vi "UndoEngine.vi"(0 "reference":refnum<class "Graph.lvclass">, 1 "Action":enum16{"TakeSnapshot", "Undo", "Redo"}(ring), 2 "Reset":bool, 3 "graphics":refnum<class "Graphics.lvclass">, 4 "grid":refnum<class "Grid.lvclass">, 5 "error in (no error)":errorcluster, 6 "menu":refnum<k9>, 8 "UndoLevels(ignoredIfNotWired)":i32=-1) -> (19 "error out":errorcluster)   [LabVIEW 2014, in "Graph.lvclass"]
doc: "Save to File"
uses:
  <resource>/Framework/Providers/Open_GDS/UML/Graph_class/Graph.lvclass
  <resource>/Framework/Providers/Open_GDS/UML/Grid_class/Grid.lvclass
  <resource>/Framework/Providers/Open_GDS/UML/Graphics_class/Graphics.lvclass
  <resource>/Framework/Providers/Open_GDS/UML/Graph_class/private/diagramType.ctl
  <resource>/Framework/Providers/Open_GDS/UML/AbstractNode_class/AbstractNode.lvclass
  <resource>/Framework/Providers/Open_GDS/UML/AbstractEdge_class/AbstractEdge.lvclass
  <resource>/Framework/Providers/Open_GDS/UML/General/Rectangle/Rectangle Rectangle2D.ctl
  <resource>/Framework/Providers/Open_GDS/UML/StateDiagramGraph_class/private/StateDiagramData.ctl
  <resource>/Framework/Providers/Open_GDS/UML/StateDiagramGraph_class/private/ViPathShowOption.ctl
  <resource>/Framework/Providers/Open_GDS/UML/ClassDiagramGraph_class/ClassDiagramGraph.lvclass
  <resource>/Framework/Providers/Open_GDS/UML/SequenceDiagramGraph_class/SequenceDiagramGraph.lvclass
  <resource>/Framework/Providers/Open_GDS/UML/UseCaseDiagramGraph_class/UseCaseDiagramGraph.lvclass
  <resource>/Framework/Providers/Open_GDS/UML/StateDiagramGraph_class/StateDiagramGraph.lvclass
  <resource>/Framework/Providers/Open_GDS/UML/PointNode_class/PointNode.lvclass
panel:
  out "error out 2":errorcluster
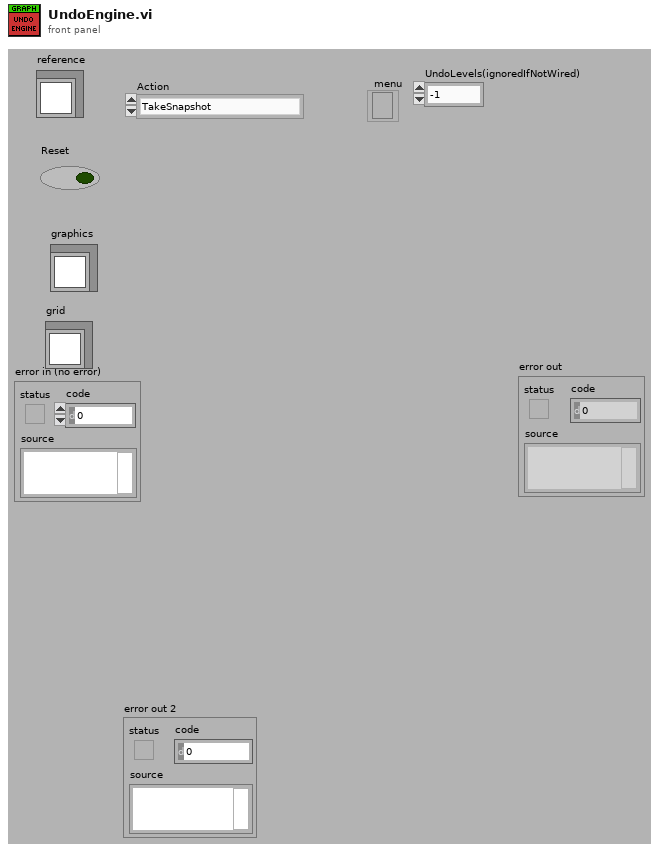
[diagram p1: front panel]
types:
  T1 = cluster{"DiagramData":string, "nodeInfo":cluster{"NodeType":string[], "ParentIndex":i32[], "ChildernIndexies":cluster{i32[]}[], "FlattenData":string[]}, "edgeInfo":cluster{"EdgeType":string[], "StartNodeIndex":i32[], "EndNodeIndex":i32[], "FlattenData":string[]}}
  T2 = cluster{"nodeInfo":cluster{"NodeType":string[], "ParentIndex":i32[], "ChildernIndexies":cluster{i32[]}[], "FlattenData":string[]}, "edgeInfo":cluster{"EdgeType":string[], "StartNodeIndex":i32[], "EndNodeIndex":i32[], "FlattenData":string[]}, "Succeeded":bool, "DiagramData":string}
  T3 = typedef "Graph.lvclass/diagramType.ctl" = enum16{"None", "Class", "Sequency", "State", "UseCase", "DQMH-Module"}
  T4 = typedef "Rectangle Rectangle2D.ctl" = cluster{"x":dbl, "y":dbl, "width":dbl, "height":dbl}
  T5 = cluster{"graph":refnum<class "Graph.lvclass">, "succeeded":bool, "diagramType":T3, "nodeInfo":cluster{"NodeType":string[], "ParentIndex":i32[], "ChildernIndexies":cluster{i32[]}[], "FlattenData":string[]}, "edgeInfo":cluster{"EdgeType":string[], "StartNodeIndex":i32[], "EndNodeIndex":i32[], "FlattenData":string[]}, "nodes":refnum<class "AbstractNode.lvclass">[], "edges":refnum<class "AbstractEdge.lvclass">[], "DiagramData":string, "bounds":T4}
  T6 = typedef "StateDiagramGraph.lvclass/StateDiagramData.ctl" = cluster{"VI-Path":path, "ShowOption":T7}
  T7 = typedef "StateDiagramGraph.lvclass/ViPathShowOption.ctl" = enum16{"Don't Show", "Show Relative Path", "Show Absolute Path"}
  T8 = cluster{"DiagramData":string, "nodeInfo":cluster{"NodeType":string[], "ParentIndex":i32[], "ChildernIndexies":cluster{i32[]}[], "FlattenData":string[]}, "edgeInfo":cluster{"EdgeType":string[], "StartNodeIndex":i32[], "EndNodeIndex":i32[], "FlattenData":string[]}}[]
  T9 = typedef "Graph.lvclass/ObjectAttributes.ctl" = cluster{"nodes":refnum<class "AbstractNode.lvclass">[], "edges":refnum<class "AbstractEdge.lvclass">[], "nodesToBeRemoved":refnum<class "AbstractNode.lvclass">[], "edgesToBeRemoved":refnum<class "AbstractEdge.lvclass">[], "needsLayout":bool, "LayoutNodes":refnum<class "AbstractNode.lvclass">[]}
  T10 = cluster{"children":refnum<class "AbstractNode.lvclass">[]}
  T11 = cluster{"NodeType":string[], "ParentIndex":i32[], "ChildernIndexies":cluster{i32[]}[], "FlattenData":string[]}
  T12 = cluster{"EdgeType":string[], "StartNodeIndex":i32[], "EndNodeIndex":i32[], "FlattenData":string[]}
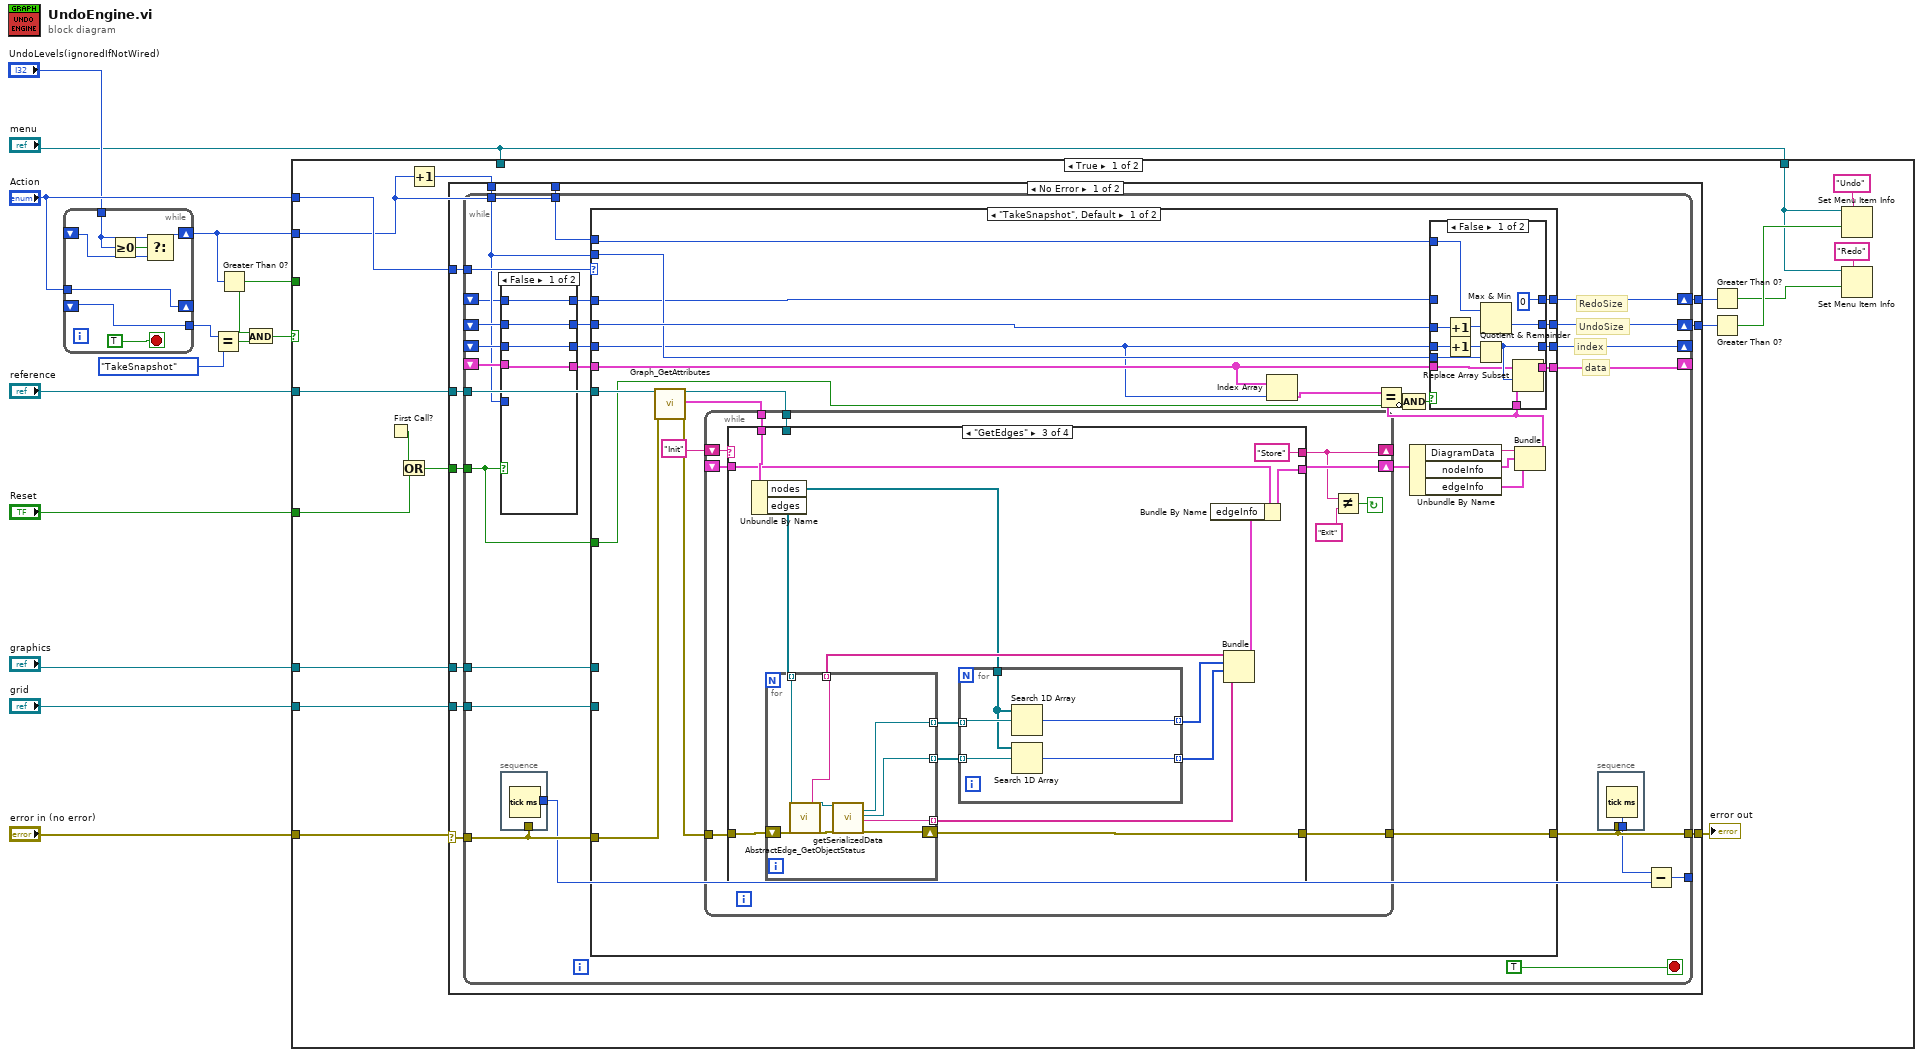
[diagram p0: block diagram]
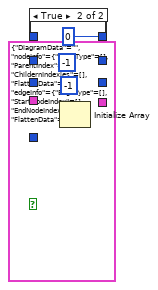
[diagram p2: hidden frame]
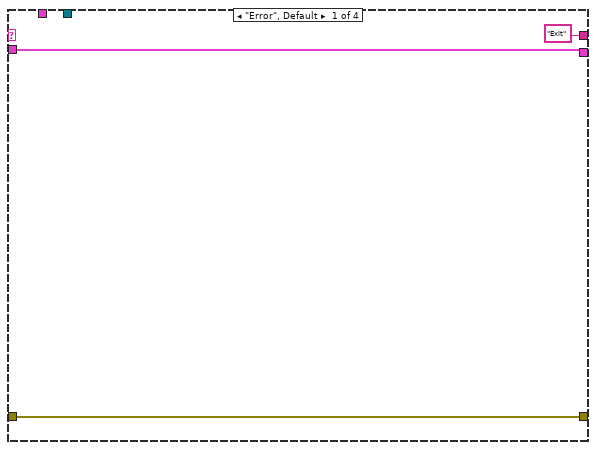
[diagram p4: hidden frame]
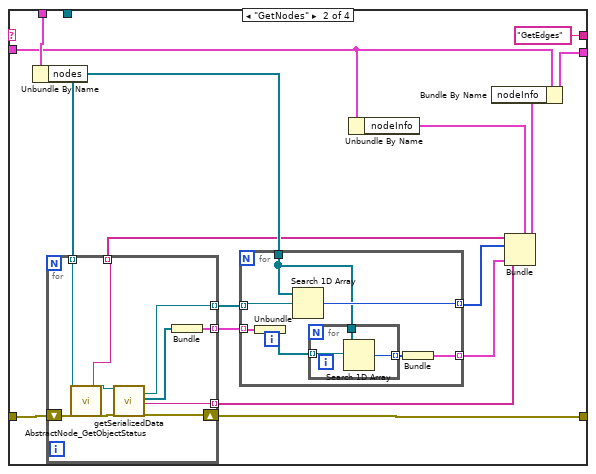
[diagram p5: hidden frame]
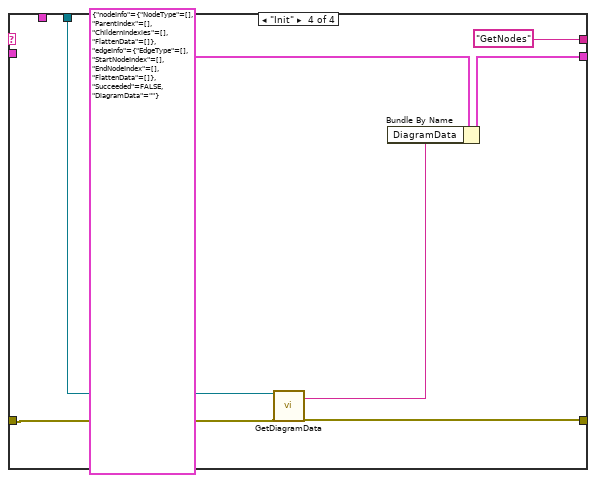
[diagram p6: hidden frame]
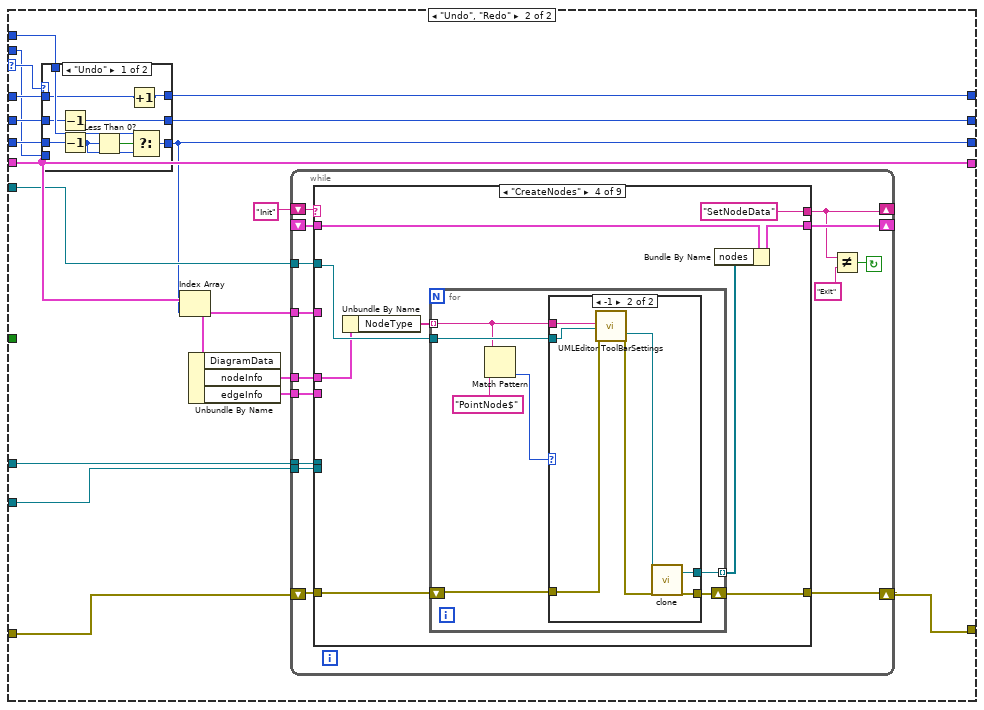
[diagram p7: hidden frame]
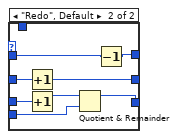
[diagram p8: hidden frame]
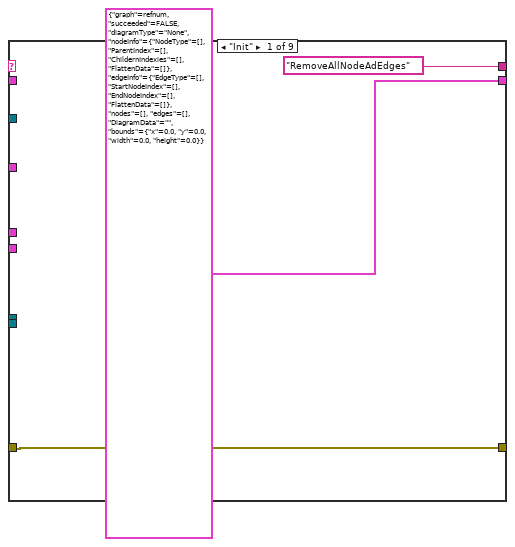
[diagram p9: hidden frame]
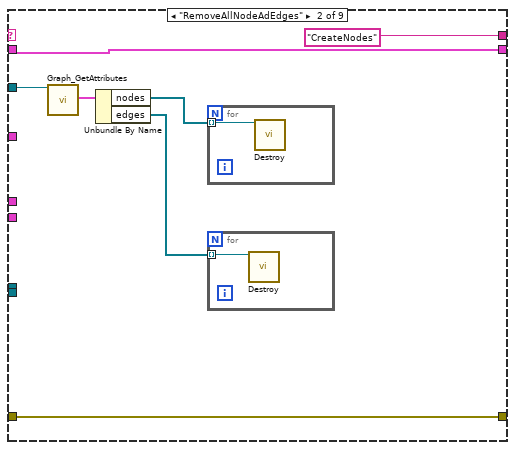
[diagram p10: hidden frame]
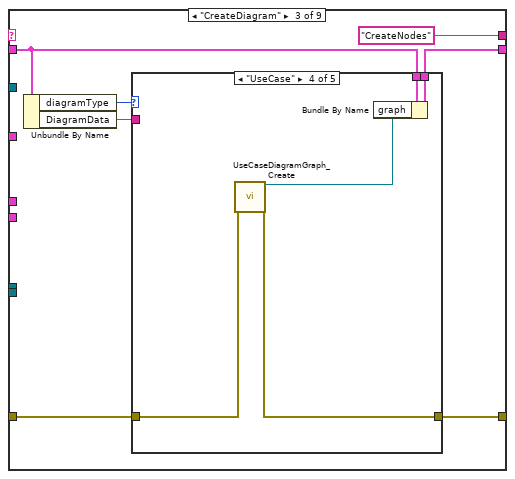
[diagram p11: hidden frame]
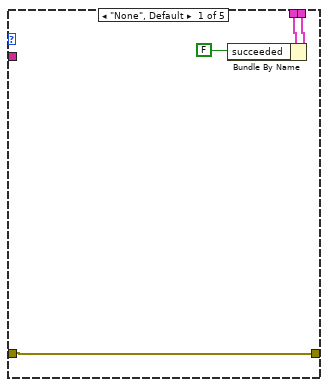
[diagram p12: hidden frame]
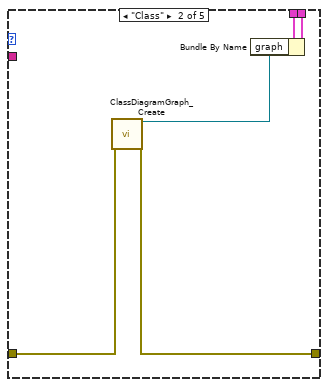
[diagram p13: hidden frame]
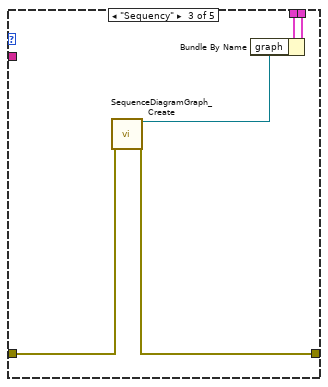
[diagram p14: hidden frame]
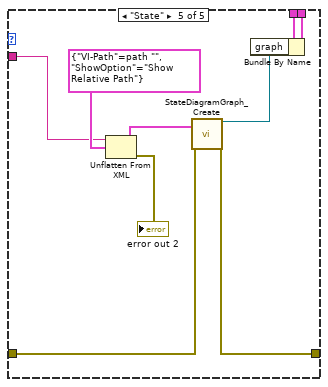
[diagram p15: hidden frame]
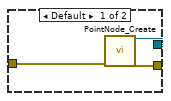
[diagram p16: hidden frame]
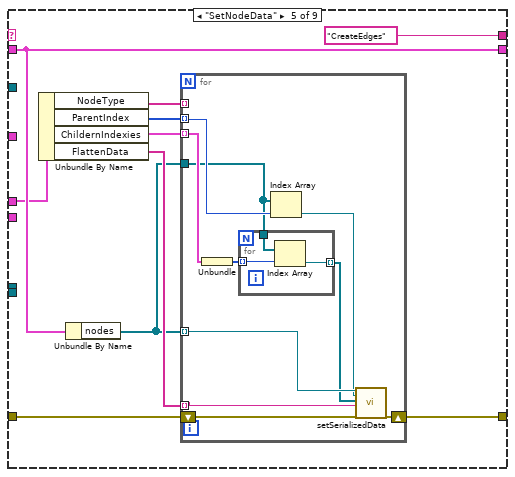
[diagram p17: hidden frame]
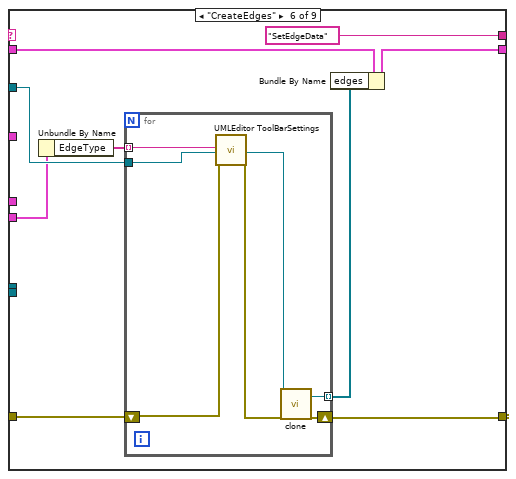
[diagram p18: hidden frame]
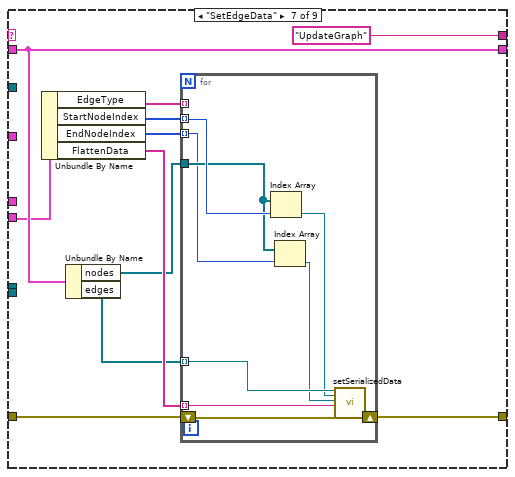
[diagram p19: hidden frame]
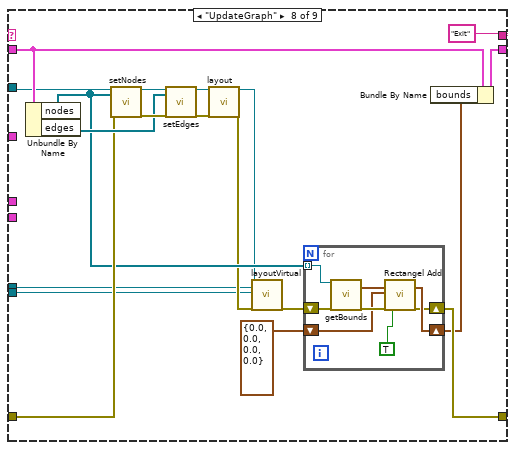
[diagram p20: hidden frame]
diagram:
  n1 = while {
    shift-right: [w19] -> _
    shift-left: _ -> [w20]
    tunnel: [w20] -> w7
    shift-right: [w15] -> w4
    shift-left: _ -> [w16]
    tunnel: "Action" -> [w19]
    tunnel: "UndoLevels(ignoredIfNotWired)" -> [w17]
    stop <- TRUE stop-if-true
    n2 = Greater Or Equal To 0?(x=w17) -> (x >= 0?=w18:bool)
    n3 = Select(t=w17, s=w18, f=w16) -> (s? t:f=w15:i32)
  }
  n4 = Equal?(x=w7, y=enum16{"TakeSnapshot", "Undo", "Redo"}."TakeSnapshot") -> (x = y?=w5:bool)
  n5 = Greater Than 0?(x=w4) -> (x > 0?=w2:bool)
  n6 = And(x=w2, y=w5) -> (x .and. y?=w3:bool)
  n7 = case shown="True" w3 {
    tunnel: "reference" -> [w39 _]
    tunnel: "error in (no error)" -> [w37 _]
    tunnel: "Reset" -> [w36 _]
    tunnel: "graphics" -> [w33 _]
    tunnel: "grid" -> [w32 _]
    tunnel: "Action" -> [w31 _]
    tunnel: w4 -> [w29 _]
    tunnel: w2 -> [_ w426]
    tunnel: "menu" -> [_ w425]
    tunnel: "menu" -> [w24 _]
    frame True {
      n8 = First Call?() -> (First Call?: T/F=w35:bool)
      n9 = Or(x=w35, y=w36) -> (x .or. y?=w34:bool)
      n10 = Increment(x=w29) -> (x+1=w30:i32)
      n11 = case shown="No Error" w37 {
        selector: w37 -> [w48 w424]
        tunnel: w39 -> [w50 _]
        tunnel: [w49 w424] -> w38
        tunnel: w31 -> [w47 _]
        tunnel: w34 -> [w46 _]
        tunnel: [w45 _] -> w22
        tunnel: w30 -> [w44 _]
        tunnel: w33 -> [w43 _]
        tunnel: w32 -> [w42 _]
        tunnel: w29 -> [w41 _]
        tunnel: [w40 _] -> w23
        frame No Error {
          n12 = while {
            tunnel: w50 -> [w75]
            tunnel: [w55] -> w49
            tunnel: w48 -> [w54]
            tunnel: w47 -> [w74]
            shift-right: [w64] -> _
            shift-left: _ -> [w69]
            shift-right: [w70] -> _
            shift-left: _ -> [w72]
            tunnel: w46 -> [w61]
            shift-right: [w65] -> w45
            shift-left: _ -> [w67]
            tunnel: w44 -> [w60]
            tunnel: w43 -> [w63]
            tunnel: w42 -> [w62]
            tunnel: w41 -> [w59]
            shift-right: [w56] -> w40
            shift-left: _ -> [w58]
            tunnel: [w51] -> _
            stop <- TRUE stop-if-true
            # "RedoSize"
            # "data"
            # "UndoSize"
            # "index"
            n13 = case shown="False" w61 {
              tunnel: w72 -> [w80 _]
              tunnel: [w80 -1] -> w71
              tunnel: w69 -> [w79 _]
              tunnel: [w79 w85] -> w68
              tunnel: w67 -> [w81 _]
              tunnel: [w81 -1] -> w66
              tunnel: w60 -> [_ w83]
              tunnel: [w78 0] -> w57
              tunnel: w58 -> [w78 _]
              frame False {
              }
              frame True {
                n14 = Initialize Array(T1 {"DiagramData"="", "nodeInfo"={"NodeType"=[], "ParentIndex"=[], "ChildernIndexies"=[], "FlattenData"=[]}, "edgeInfo"={"EdgeType"=[], "StartNodeIndex"=[], "EndNodeIndex"=[], "FlattenData"=[]}} ("output cluster"), w83) -> (w85:T8)
              }
            }
            n15 = stacked-sequence {
              tunnel: w54 -> [_]
              tunnel: [w76] -> w52
              frame #0 {
                n16 = Tick Count (ms)() -> (millisecond timer value=w76:u32)
              }
            }
            n17 = case shown="\"TakeSnapshot\", Default" w74 {
              selector: w74 -> [_ w219]
              tunnel: w75 -> [w113 w227]
              tunnel: [w112 w225] -> w55
              tunnel: w54 -> [w89 w226]
              tunnel: w71 -> [w98 w230]
              tunnel: [w102 w222] -> w70
              tunnel: w68 -> [w99 w228]
              tunnel: w66 -> [w104 w221]
              tunnel: [w100 w229] -> w65
              tunnel: w60 -> [w101 w213]
              tunnel: [w103 w228] -> w64
              tunnel: w63 -> [_ w224]
              tunnel: w62 -> [_ w223]
              tunnel: w61 -> [w93 _]
              tunnel: w59 -> [w91 w212]
              tunnel: w57 -> [w90 w218]
              tunnel: [w92 w220] -> w56
              frame "TakeSnapshot", Default {
                n18 = call <resource>:"Graph_GetAttributes.vi"("reference in"=w113, "error in (no error)"=w89) -> ("reference out"=w111:refnum<class "Graph.lvclass">, "Data"=w88:T9, "error out"=w110:errorcluster)  [unwired: 1 in, 14 out]
                n19 = while {
                  tunnel: w88 -> [w139]
                  tunnel: w110 -> [w138]
                  tunnel: [w137] -> w112
                  shift-right: [w132] -> _
                  shift-left: "Init" -> [w136]
                  shift-right: [w135] -> w108
                  shift-left: _ -> [w131]
                  tunnel: w111 -> [w130]
                  stop <- w133 continue-if-true
                  n20 = case shown="\"GetEdges\"" w136 {
                    tunnel: w139 -> [_ w157 w191 _]
                    tunnel: w138 -> [w142 w156 w190 w208]
                    tunnel: [w142 w150 w177 w207] -> w137
                    tunnel: [w140 w146 w183 w209] -> w135
                    tunnel: ["Exit" ("y") "GetEdges" "Store" "GetNodes"] -> w132
                    tunnel: w131 -> [w140 w144 w185 _]
                    tunnel: w130 -> [_ _ _ w205]
                    frame "Error", Default {
                    }
                    frame "GetNodes" {
                      n21 = Unbundle By Name(w157) -> ("nodes"=w149:refnum<class "AbstractNode.lvclass">[])
                      n22 = for {
                        shift-right: [w169] -> w150
                        shift-left: w156 -> [w176]
                        tunnel: w149 -> [w172] mode=indexing
                        tunnel: [w175] -> w155 mode=indexing
                        tunnel: [w173] -> w154 mode=indexing
                        tunnel: [w170] -> w151 mode=indexing
                        tunnel: [w168] -> w148 mode=indexing
                        n23 = call <resource>:"AbstractNode_GetObjectStatus.vi"("reference in"=w172) -> ("Class name"=w168:string, "reference out"=w171:refnum<class "AbstractNode.lvclass">)  [unwired: 1 in, 16 out]
                        n24 = call-dynamic "getSerializedData.vi"("reference"=w171, "error in (no error)"=w176) -> ("parent"=w175:refnum<class "AbstractNode.lvclass">, "children"=w174:refnum<class "AbstractNode.lvclass">[], "xmlOut"=w170:string, "error out"=w169:errorcluster)  [unwired: 13 in, 1 out]
                        n25 = Bundle("children"=w174) -> (w173:T10)  [unwired: 1 in]
                      }
                      n26 = for {
                        tunnel: w155 -> [w163] mode=indexing
                        tunnel: w154 -> [w164] mode=indexing
                        tunnel: [w162] -> w153 mode=indexing
                        tunnel: [w159] -> w152 mode=indexing
                        tunnel: w149 -> [w158]
                        n27 = Unbundle(w164) -> ("children"=w161:refnum<class "AbstractNode.lvclass">[])
                        n28 = Search 1D Array(1D array=w158, element=w163) -> (index of element=w162:i32)  [unwired: 1 out]
                        n29 = for {
                          tunnel: w161 -> [w166] mode=indexing
                          tunnel: w158 -> [w167]
                          tunnel: [w165] -> w160 mode=indexing
                          n30 = Search 1D Array(1D array=w167, element=w166) -> (index of element=w165:i32)  [unwired: 1 out]
                        }
                        n31 = Bundle(w160) -> (w159:cluster{i32[]})  [unwired: 1 in]
                      }
                      n32 = Unbundle By Name(w144) -> ("nodeInfo"=w143:T11)
                      n33 = Bundle(cluster=w143, "NodeType"=w148, "ParentIndex"=w153, "ChildernIndexies"=w152, "FlattenData"=w151) -> (w147:T11)
                      n34 = Bundle By Name(cluster=w144, "nodeInfo"=w147) -> (w146:T2)
                    }
                    frame "GetEdges" {
                      n35 = Unbundle By Name(w191) -> ("nodes"=w181:refnum<class "AbstractNode.lvclass">[], "edges"=w180:refnum<class "AbstractEdge.lvclass">[])
                      n36 = for {
                        shift-right: [w198] -> w177
                        shift-left: w190 -> [w204]
                        tunnel: w180 -> [w202] mode=indexing
                        tunnel: [w203] -> w189 mode=indexing
                        tunnel: [w199] -> w187 mode=indexing
                        tunnel: [w197] -> w186 mode=indexing
                        tunnel: [w200] -> w179 mode=indexing
                        n37 = call <resource>:"AbstractEdge_GetObjectStatus.vi"("reference in"=w202) -> ("Class name"=w197:string, "reference out"=w201:refnum<class "AbstractEdge.lvclass">)  [unwired: 1 in, 16 out]
                        n38 = call-dynamic "getSerializedData.vi"("reference"=w201, "error in (no error)"=w204) -> ("startNode"=w203:refnum<class "AbstractNode.lvclass">, "endNode"=w200:refnum<class "AbstractNode.lvclass">, "xmlOut"=w199:string, "error out"=w198:errorcluster)  [unwired: 13 in, 1 out]
                      }
                      n39 = for {
                        tunnel: w189 -> [w196] mode=indexing
                        tunnel: [w195] -> w188 mode=indexing
                        tunnel: w181 -> [w194]
                        tunnel: w179 -> [w193] mode=indexing
                        tunnel: [w192] -> w178 mode=indexing
                        n40 = Search 1D Array(1D array=w194, element=w196) -> (index of element=w195:i32)  [unwired: 1 out]
                        n41 = Search 1D Array(1D array=w194, element=w193) -> (index of element=w192:i32)  [unwired: 1 out]
                      }
                      n42 = Bundle(w186, w188, w178, w187) -> (w184:cluster{string[], i32[], i32[], string[]})  [unwired: 1 out]
                      n43 = Bundle By Name(cluster=w185, "edgeInfo"=w184) -> (w183:T2)
                    }
                    frame "Init" {
                      n44 = call-dynamic "GetDiagramData.vi"("reference"=w205, "error in (no error)"=w208) -> ("DiagramData"=w206:string, "error out"=w207:errorcluster)  [unwired: 15 in, 1 out]
                      n45 = Bundle By Name(cluster=T2 {"nodeInfo"={"NodeType"=[], "ParentIndex"=[], "ChildernIndexies"=[], "FlattenData"=[]}, "edgeInfo"={"EdgeType"=[], "StartNodeIndex"=[], "EndNodeIndex"=[], "FlattenData"=[]}, "Succeeded"=FALSE, "DiagramData"=""}, "DiagramData"=w206) -> (w209:T2)
                    }
                  }
                  n46 = Not Equal?(x=w132, y="Exit") -> (x != y?=w133:bool)
                }
                n47 = Index Array(array=w99, index=w98) -> (element=w96:T1)
                n48 = Unbundle By Name(w108) -> ("DiagramData"=w107:string, "nodeInfo"=w106:T11, "edgeInfo"=w105:T12)
                n49 = Bundle("DiagramData"=w107, "nodeInfo"=w106, "edgeInfo"=w105) -> (w97:T1)  [unwired: 1 out]
                n50 = Equal?(x=w96, y=w97) -> (x = y?=w95:bool)
                n51 = Compound Arithmetic op=AND(w95, invert w93) -> (w94:bool)
                n52 = case shown="False" w94 {
                  tunnel: w104 -> [w125 w129]
                  tunnel: [w123 w127] -> w103
                  tunnel: [w122 w128] -> w102
                  tunnel: w101 -> [w115 _]
                  tunnel: [w120 w129] -> w100
                  tunnel: w99 -> [w119 w127]
                  tunnel: w98 -> [w118 w128]
                  tunnel: w97 -> [w117 _]
                  tunnel: w91 -> [w116 _]
                  tunnel: [0 w126] -> w92
                  tunnel: w90 -> [_ w126]
                  frame False {
                    n53 = Increment(x=w125) -> (x+1=w121:i32)
                    n54 = Increment(x=w118) -> (x+1=w124:i32)
                    n55 = Quotient & Remainder(x=w124, y=w115) -> (x-y*floor(x/y)=w122:i32)  [unwired: 1 out]
                    n56 = Max & Min(x=w116, y=w121) -> (min(x,y)=w120:i32)  [unwired: 1 out]
                    n57 = Replace Array Subset(array=w119, new element=w117, index=w122) -> (w123:T8)
                  }
                  frame True {
                  }
                }
              }
              frame "Undo", "Redo" {
                n58 = case shown="\"Undo\"" w219 {
                  tunnel: w230 -> [w239 w247]
                  tunnel: [w238 w246] -> w229
                  tunnel: w212 -> [w235 _]
                  tunnel: [w234 w241] -> w222
                  tunnel: w221 -> [w233 w245]
                  tunnel: w218 -> [w232 w244]
                  tunnel: [w231 w243] -> w220
                  tunnel: w213 -> [_ w240]
                  frame "Undo" {
                    n59 = Decrement(x=w233) -> (x-1=w238:i32)
                    n60 = Decrement(x=w239) -> (x-1=w236:i32)
                    n61 = Less Than 0?(x=w236) -> (x < 0?=w237:bool)
                    n62 = Increment(x=w232) -> (x+1=w231:i32)
                    n63 = Select(t=w235, s=w237, f=w236) -> (s? t:f=w234:i32)
                  }
                  frame "Redo", Default {
                    n64 = Increment(x=w245) -> (x+1=w246:i32)
                    n65 = Increment(x=w247) -> (x+1=w242:i32)
                    n66 = Quotient & Remainder(x=w242, y=w240) -> (x-y*floor(x/y)=w241:i32)  [unwired: 1 out]
                    n67 = Decrement(x=w244) -> (x-1=w243:i32)
                  }
                }
                n68 = Index Array(array=w228, index=w222) -> (element=w216:T1)
                n69 = Unbundle By Name(w216) -> ("nodeInfo"=w215:T11, "edgeInfo"=w214:T12)  [unwired: 1 out]
                n70 = while {
                  shift-right: [w257] -> _
                  shift-left: "Init" -> [w261]
                  shift-right: [w260] -> _
                  shift-left: _ -> [w256]
                  shift-right: [w254] -> w225
                  shift-left: w226 -> [w255]
                  tunnel: w224 -> [w253]
                  tunnel: w223 -> [w252]
                  tunnel: w216 -> [w251]
                  tunnel: w227 -> [w250]
                  tunnel: w215 -> [w249]
                  tunnel: w214 -> [w248]
                  stop <- w258 continue-if-true
                  n71 = case shown="\"CreateNodes\"" w261 {
                    tunnel: w255 -> [w264 w271 w276 w315 w339 w364 w379 w407 w423]
                    tunnel: [w264 w271 w275 w311 w338 w361 w378 w402 w423] -> w254
                    tunnel: [T5 {"graph"=refnum, "succeeded"=FALSE, "diagramType"=enum."None", "nodeInfo"={"NodeType"=[], "ParentIndex"=[], "ChildernIndexies"=[], "FlattenData"=[]}, "edgeInfo"={"EdgeType"=[], "StartNodeIndex"=[], "EndNodeIndex"=[], "FlattenData"=[]}, "nodes"=[], "edges"=[], "DiagramData"="", "bounds"={"x"=0.0, "y"=0.0, "width"=0.0, "height"=0.0}} ("localData") w267 w278 w313 w337 w363 w377 w405 w421] -> w260
                    tunnel: ["RemoveAllNodeAdEdges" "CreateNodes" "CreateNodes" "SetNodeData" "CreateEdges" ("y") "SetEdgeData" "UpdateGraph" ("y") "Exit" ("y") "Exit" ("y")] -> w257
                    tunnel: w256 -> [_ w267 w277 w312 w337 w362 w377 w404 w421]
                    tunnel: w253 -> [_ _ _ _ _ _ _ w396 _]
                    tunnel: w252 -> [_ _ _ _ _ _ _ w395 _]
                    tunnel: w251 -> [_ _ _ _ _ _ _ _ _]
                    tunnel: w250 -> [_ w270 _ w310 _ w359 _ w394 _]
                    tunnel: w249 -> [_ _ _ w309 w335 _ _ _ _]
                    tunnel: w248 -> [_ _ _ _ _ w358 w374 _ _]
                    frame "Init" {
                    }
                    frame "RemoveAllNodeAdEdges" {
                      n72 = call <resource>:"Graph_GetAttributes.vi"("reference in"=w270) -> ("Data"=w265:T9)  [unwired: 2 in, 16 out]
                      n73 = Unbundle By Name(w265) -> ("nodes"=w269:refnum<class "AbstractNode.lvclass">[], "edges"=w268:refnum<class "AbstractEdge.lvclass">[])
                      n74 = for {
                        tunnel: w269 -> [w273] mode=indexing
                        n75 = call-dynamic "Destroy.vi"("reference"=w273) -> ()  [unwired: 17 in, 2 out]
                      }
                      n76 = for {
                        tunnel: w268 -> [w272] mode=indexing
                        n77 = call-dynamic "Destroy.vi"("reference"=w272) -> ()  [unwired: 18 in, 1 out]
                      }
                    }
                    frame "CreateDiagram" {
                      n78 = Unbundle By Name(w277) -> ("diagramType"=w279:T3, "DiagramData"=w274:string)
                      n79 = case shown="\"UseCase\"" w279 {
                        tunnel: w277 -> [w284 w289 w294 w299 w308]
                        tunnel: [w283 w288 w293 w298 w307] -> w278
                        tunnel: w276 -> [w281 w287 w292 w297 w306]
                        tunnel: [w281 w286 w291 w296 w305] -> w275
                        tunnel: w274 -> [_ _ _ _ w300]
                        frame "None", Default {
                          n80 = Bundle By Name(cluster=w284, "succeeded"=FALSE) -> (w283:T5)
                        }
                        frame "Class" {
                          n81 = call <resource>:"ClassDiagramGraph_Create.vi"("error in (no error)"=w287) -> ("reference out"=w285:refnum<class "ClassDiagramGraph.lvclass">, "error out"=w286:errorcluster)  [unwired: 1 in, 16 out]
                          n82 = Bundle By Name(cluster=w289, "graph"=w285) -> (w288:T5)
                        }
                        frame "Sequency" {
                          n83 = call <resource>:"SequenceDiagramGraph_Create.vi"("error in (no error)"=w292) -> ("reference out"=w290:refnum<class "SequenceDiagramGraph.lvclass">, "error out"=w291:errorcluster)  [unwired: 1 in, 16 out]
                          n84 = Bundle By Name(cluster=w294, "graph"=w290) -> (w293:T5)
                        }
                        frame "UseCase" {
                          n85 = call <resource>:"UseCaseDiagramGraph_Create.vi"("error in (no error)"=w297) -> ("reference out"=w295:refnum<class "UseCaseDiagramGraph.lvclass">, "error out"=w296:errorcluster)  [unwired: 1 in, 16 out]
                          n86 = Bundle By Name(cluster=w299, "graph"=w295) -> (w298:T5)
                        }
                        frame "State" {
                          n87 = Unflatten From XML(xml string=w300, type=T6 {"VI-Path"=path "", "ShowOption"=enum."Show Relative Path"} ("StateDiagramData")) -> (value=w303:T6, error out=→"error out 2":errorcluster)  [unwired: 1 in]
                          n88 = call <resource>:"StateDiagramGraph_Create.vi"("StateDiagramData"=w303, "error in (no error)"=w306) -> ("reference out"=w304:refnum<class "StateDiagramGraph.lvclass">, "error out"=w305:errorcluster)  [unwired: 1 in, 15 out]
                          n89 = Bundle By Name(cluster=w308, "graph"=w304) -> (w307:T5)
                        }
                      }
                    }
                    frame "CreateNodes" {
                      n90 = Unbundle By Name(w309) -> ("NodeType"=w316:string[])
                      n91 = for {
                        tunnel: w316 -> [w318] mode=indexing
                        shift-right: [w321] -> w311
                        shift-left: w315 -> [w323]
                        tunnel: [w324] -> w314 mode=indexing
                        tunnel: w310 -> [w322]
                        n92 = Match Pattern(string=w318, regular expression="PointNode$") -> (offset past match=w319:i32)  [unwired: 4 out]
                        n93 = case shown="-1" w319 {
                          tunnel: [w326 w334] -> w324
                          tunnel: w318 -> [_ w333]
                          tunnel: w323 -> [w327 w332]
                          tunnel: w322 -> [_ w330]
                          tunnel: [w325 w328] -> w321
                          frame Default {
                            n94 = call <resource>:"PointNode_Create.vi"("error in (no error)"=w327) -> ("reference out"=w326:refnum<class "PointNode.lvclass">, "error out"=w325:errorcluster)  [unwired: 1 in, 16 out]
                          }
                          frame -1 {
                            n95 = call <resource>:"UMLEditor ToolBarSettings.vi"("NodeName/EdgeName(empty=not in use)"=w333, "graph(only used with className input)"=w330, "error in (no error)"=w332) -> ("prototypeNode"=w329:refnum<class "AbstractNode.lvclass">, "error out"=w331:errorcluster)  [unwired: 1 in, 14 out]
                            n96 = call-dynamic "clone.vi"("reference"=w329, "error in (no error)"=w331) -> ("clonedAbstractNode"=w334:refnum<class "AbstractNode.lvclass">, "error out"=w328:errorcluster)  [unwired: 15 in, 1 out]
                          }
                        }
                      }
                      n97 = Bundle By Name(cluster=w312, "nodes"=w314) -> (w313:T5)
                    }
                    frame "SetNodeData" {
                      n98 = Unbundle By Name(w335) -> ("NodeType"=w343:string[], "ParentIndex"=w342:i32[], "ChildernIndexies"=w341:cluster{i32[]}[], "FlattenData"=w340:string[])
                      n99 = Unbundle By Name(w337) -> ("nodes"=w336:refnum<class "AbstractNode.lvclass">[])
                      n100 = for {
                        tunnel: w343 -> [_] mode=indexing
                        tunnel: w342 -> [w354] mode=indexing
                        tunnel: w341 -> [w353] mode=indexing
                        tunnel: w336 -> [w352]
                        tunnel: w336 -> [w350] mode=indexing
                        tunnel: w340 -> [w346] mode=indexing
                        shift-right: [w347] -> w338
                        shift-left: w339 -> [w345]
                        n101 = Unbundle(w353) -> (w351:i32[])
                        n102 = for {
                          tunnel: w352 -> [w357]
                          tunnel: w351 -> [w356] mode=indexing
                          tunnel: [w355] -> w348 mode=indexing
                          n103 = Index Array(array=w357, index=w356) -> (element=w355:refnum<class "AbstractNode.lvclass">)
                        }
                        n104 = Index Array(array=w352, index=w354) -> (element=w349:refnum<class "AbstractNode.lvclass">)
                        n105 = call-dynamic "setSerializedData.vi"("reference"=w350, "parent"=w349, "children"=w348, "xmlOut"=w346, "error in (no error)"=w345) -> ("error out"=w347:errorcluster)  [unwired: 13 in, 1 out]
                      }
                    }
                    frame "CreateEdges" {
                      n106 = Unbundle By Name(w358) -> ("EdgeType"=w365:string[])
                      n107 = for {
                        tunnel: w365 -> [w372] mode=indexing
                        shift-right: [w373] -> w361
                        shift-left: w364 -> [w371]
                        tunnel: w359 -> [w369]
                        tunnel: [w367] -> w360 mode=indexing
                        n108 = call <resource>:"UMLEditor ToolBarSettings.vi"("NodeName/EdgeName(empty=not in use)"=w372, "graph(only used with className input)"=w369, "error in (no error)"=w371) -> ("prototypeEdge"=w368:refnum<class "AbstractEdge.lvclass">, "error out"=w370:errorcluster)  [unwired: 1 in, 14 out]
                        n109 = call-dynamic "clone.vi"("reference"=w368, "error in (no error)"=w370) -> ("clonedEdge"=w367:refnum<class "AbstractEdge.lvclass">, "error out"=w373:errorcluster)  [unwired: 15 in, 1 out]
                      }
                      n110 = Bundle By Name(cluster=w362, "edges"=w360) -> (w363:T5)
                    }
                    frame "SetEdgeData" {
                      n111 = Unbundle By Name(w374) -> ("EdgeType"=w383:string[], "StartNodeIndex"=w382:i32[], "EndNodeIndex"=w381:i32[], "FlattenData"=w380:string[])
                      n112 = Unbundle By Name(w377) -> ("nodes"=w376:refnum<class "AbstractNode.lvclass">[], "edges"=w375:refnum<class "AbstractEdge.lvclass">[])
                      n113 = for {
                        tunnel: w383 -> [_] mode=indexing
                        tunnel: w382 -> [w393] mode=indexing
                        tunnel: w381 -> [w387] mode=indexing
                        tunnel: w376 -> [w392]
                        tunnel: w375 -> [w391] mode=indexing
                        tunnel: w380 -> [w386] mode=indexing
                        shift-right: [w388] -> w378
                        shift-left: w379 -> [w385]
                        n114 = Index Array(array=w392, index=w393) -> (element=w390:refnum<class "AbstractNode.lvclass">)
                        n115 = Index Array(array=w392, index=w387) -> (element=w389:refnum<class "AbstractNode.lvclass">)
                        n116 = call-dynamic "setSerializedData.vi"("reference"=w391, "startNode"=w390, "endNode"=w389, "xmlOut"=w386, "error in (no error)"=w385) -> ("error out"=w388:errorcluster)  [unwired: 13 in, 1 out]
                      }
                    }
                    frame "UpdateGraph" {
                      n117 = Unbundle By Name(w404) -> ("nodes"=w401:refnum<class "AbstractNode.lvclass">[], "edges"=w410:refnum<class "AbstractEdge.lvclass">[])
                      n118 = call-dynamic "setNodes.vi"("reference"=w394, "nodes"=w401, "error in (no error)"=w407) -> ("reference out"=w412:refnum<class "Graph.lvclass">, "error out"=w411:errorcluster)  [unwired: 15 in]
                      n119 = call-dynamic "setEdges.vi"("reference"=w412, "edges"=w410, "error in (no error)"=w411) -> ("reference out"=w409:refnum<class "Graph.lvclass">, "error out"=w408:errorcluster)  [unwired: 15 in]
                      n120 = call-dynamic "layout.vi"("reference"=w409, "error in (no error)"=w408) -> ("reference out"=w398:refnum<class "Graph.lvclass">, "error out"=w397:errorcluster)  [unwired: 16 in]
                      n121 = call <resource>:"layoutVirtual.vi"("reference"=w398, "graphics"=w396, "grid"=w395, "error in (no error)"=w397) -> ("error out"=w399:errorcluster)  [unwired: 15 out]
                      n122 = for {
                        shift-right: [w415] -> w402
                        shift-left: w399 -> [w414]
                        shift-right: [w416] -> w400
                        shift-left: T4 {"x"=0.0, "y"=0.0, "width"=0.0, "height"=0.0} ("boundsAdded") -> [w417]
                        tunnel: w401 -> [w413] mode=indexing
                        n123 = call-dynamic "getBounds.vi"("reference"=w413, "error in (no error)"=w414) -> ("bounds"=w420:T4, "error out"=w419:errorcluster)  [unwired: 15 in, 1 out]
                        n124 = call <resource>:"Rectangel Add.vi"("bounds1"=w420, "bounds2"=w417, "error in (no error)"=w419, "useAbsoluteCordinates(False)"=TRUE) -> ("boundsAdded"=w416:T4, "error out"=w415:errorcluster)  [unwired: 1 in, 13 out]
                      }
                      n125 = Bundle By Name(cluster=w404, "bounds"=w400) -> (w405:T5)
                    }
                    frame "Error", Default {
                    }
                  }
                  n126 = Not Equal?(x=w257, y="Exit") -> (x != y?=w258:bool)
                }
              }
            }
            n127 = stacked-sequence {
              tunnel: w55 -> [_]
              tunnel: [w77] -> w53
              frame #0 {
                n128 = Tick Count (ms)() -> (millisecond timer value=w77:u32)
              }
            }
            n129 = Subtract(x=w53, y=w52) -> (x-y=w51:u32)
          }
        }
        frame Error {
        }
      }
      "error out" <- w38
      n130 = Greater Than 0?(x=w23) -> (x > 0?=w25:bool)
      n131 = Greater Than 0?(x=w22) -> (x > 0?=w27:bool)
      n132 = Set Menu Item Info(7:"Undo" ("item tag"), 9:w27, 11:w24) -> ()  [unwired: 1 in, 5 out]
      n133 = Set Menu Item Info(7:"Redo" ("item tag"), 9:w25, 11:w24) -> ()  [unwired: 1 in, 5 out]
    }
    frame False {
      n134 = case shown="False" w426 {
        tunnel: w425 -> [w427 _]
        frame False {
          w428 = FALSE
          n135 = Set Menu Item Info(7:"Undo" ("item tag"), 9:w428, 11:w427) -> ()  [unwired: 1 in, 5 out]
          n136 = Set Menu Item Info(7:"Redo" ("item tag"), 9:w428, 11:w427) -> ()  [unwired: 1 in, 5 out]
        }
        frame True {
        }
      }
    }
  }
